vi "ex2_4.vi"() -> ()   [LabVIEW 2017]
uses:
  <vilib>/Waveform/WDTOps.llb/WDT Append Waveforms DBL.vi
panel:
  out "DIODE VI CHARACTERISTICS":cluster{"Y":dbl[], "Y":dbl[]}[](graph)
  out "Waveform Chart":waveform(dbl)(graph)
  out "i":dbl
  out "iteration":dbl
  in  "Step size":sgl
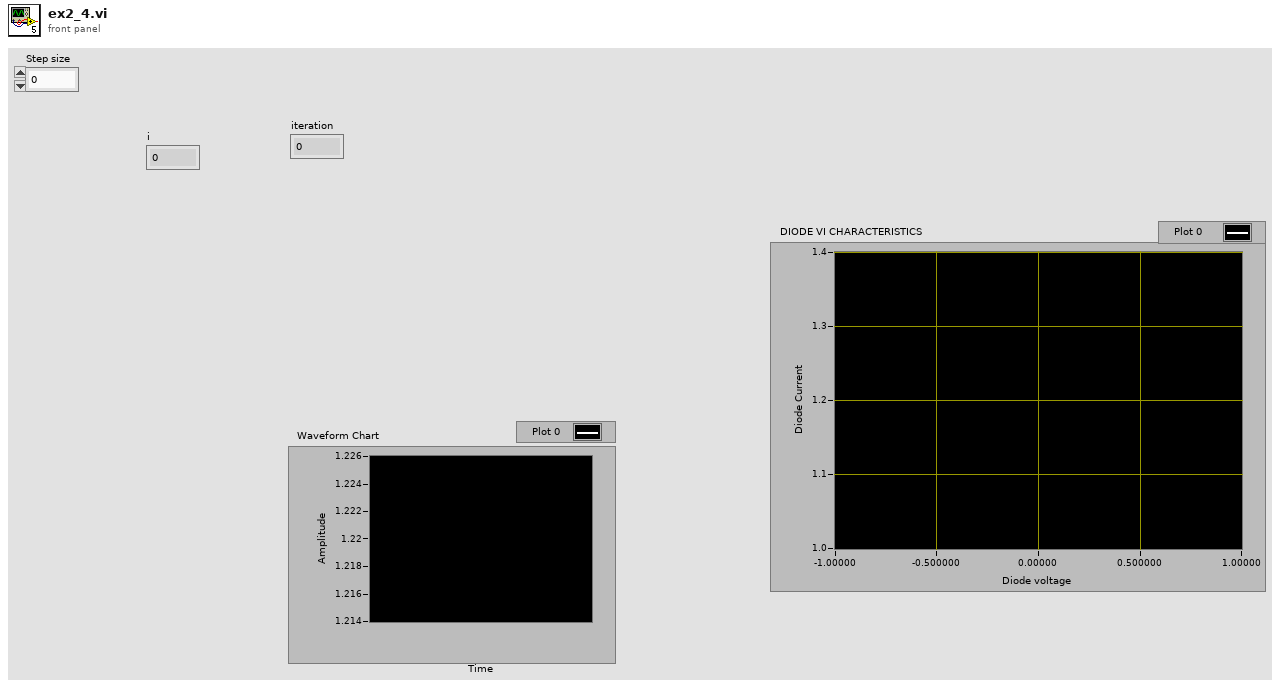
[diagram p1: front panel]
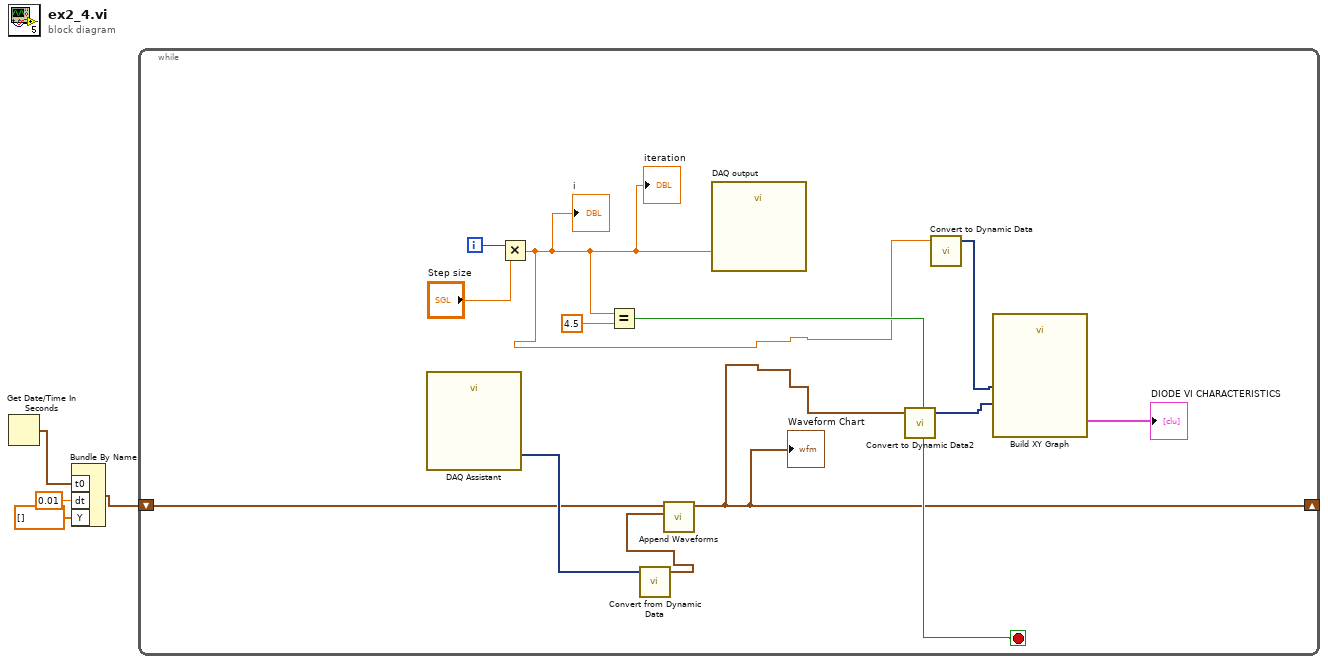
[diagram p0: block diagram]
diagram:
  n1 = Get Date/Time In Seconds() -> (seconds since 1Jan1904=w3:timestamp)
  n2 = Bundle By Name("t0"=w3, "dt"=0.01, "Y"=dbl[] []) -> (w4:waveform(dbl))  [unwired: 1 in]
  n3 = while {
    shift-right: [w6] -> _
    shift-left: w4 -> [w10]
    i -> [w16]
    stop <- w13 stop-if-true
    n4 = call "DAQ Assistant"() -> ("data"=w11:dynamicdata)  [unwired: 17 in, 2 out]
    n5 = Multiply(x=w16, y="Step size") -> (x*y=w8:sgl)
    "iteration" <- w8
    "i" <- w8
    n6 = Equal?(x=w8, y=4.5) -> (x = y?=w13:bool)
    n7 = call "Convert from Dynamic Data"("Dynamic Data Type"=w11) -> ("Waveform"=w12:waveform(dbl))  [unwired: 3 in]
    n8 = call-poly <vilib>:"Append Waveforms.vi"("waveform B"=w12, "waveform A"=w10) -> ("waveform out"=w6:waveform(dbl))  [unwired: 8 in, 1 out]
    "Waveform Chart" <- w6
    n9 = call "DAQ output"("data"=w8) -> ()  [unwired: 17 in, 2 out]
    n10 = call "Convert to Dynamic Data2"("Double"=w6) -> ("Dynamic Data Type"=w5:dynamicdata)  [unwired: 3 in]
    n11 = call "Convert to Dynamic Data"("Double"=w8) -> ("Dynamic Data Type"=w7:dynamicdata)  [unwired: 3 in]
    n12 = call "Build XY Graph"("Y Input"=w5, "X Input"=w7) -> ("XY Graph"=→"DIODE VI CHARACTERISTICS":cluster{"X":dbl[], "Y":dbl[]}[])  [unwired: 8 in, 1 out]
  }
